vi "generate_avg.vi"(4 "Summed/Average":u16, 5 "C2 enabled":bool=TRUE caption="Enabled?", 6 "Trace numer":i32=1, 7 "C1 enabled":bool=TRUE caption="Enabled?", 11 "scope Q data":T1) -> ()   [LabVIEW 2023]
uses:
  <vilib>/Waveform/WDTOps.llb/WDT Align Waveform Timestamps DBL.vi
  <vilib>/Waveform/WDTFileIO.llb/Export Waveform To Spreadsheet File.vi
  <vilib>/regexp/Match Regular Expression.xnode
panel:
  out "Channel 2 summed":waveform(dbl)(graph)
  in  "waveforms out 2":waveform(dbl)[](array[waveform])
  out "Channel 2 RT avg":waveform(dbl)(graph)
  out "Channel 1 summed":waveform(dbl)(graph)
  out "Channel 1 RT avg":waveform(dbl)(graph)
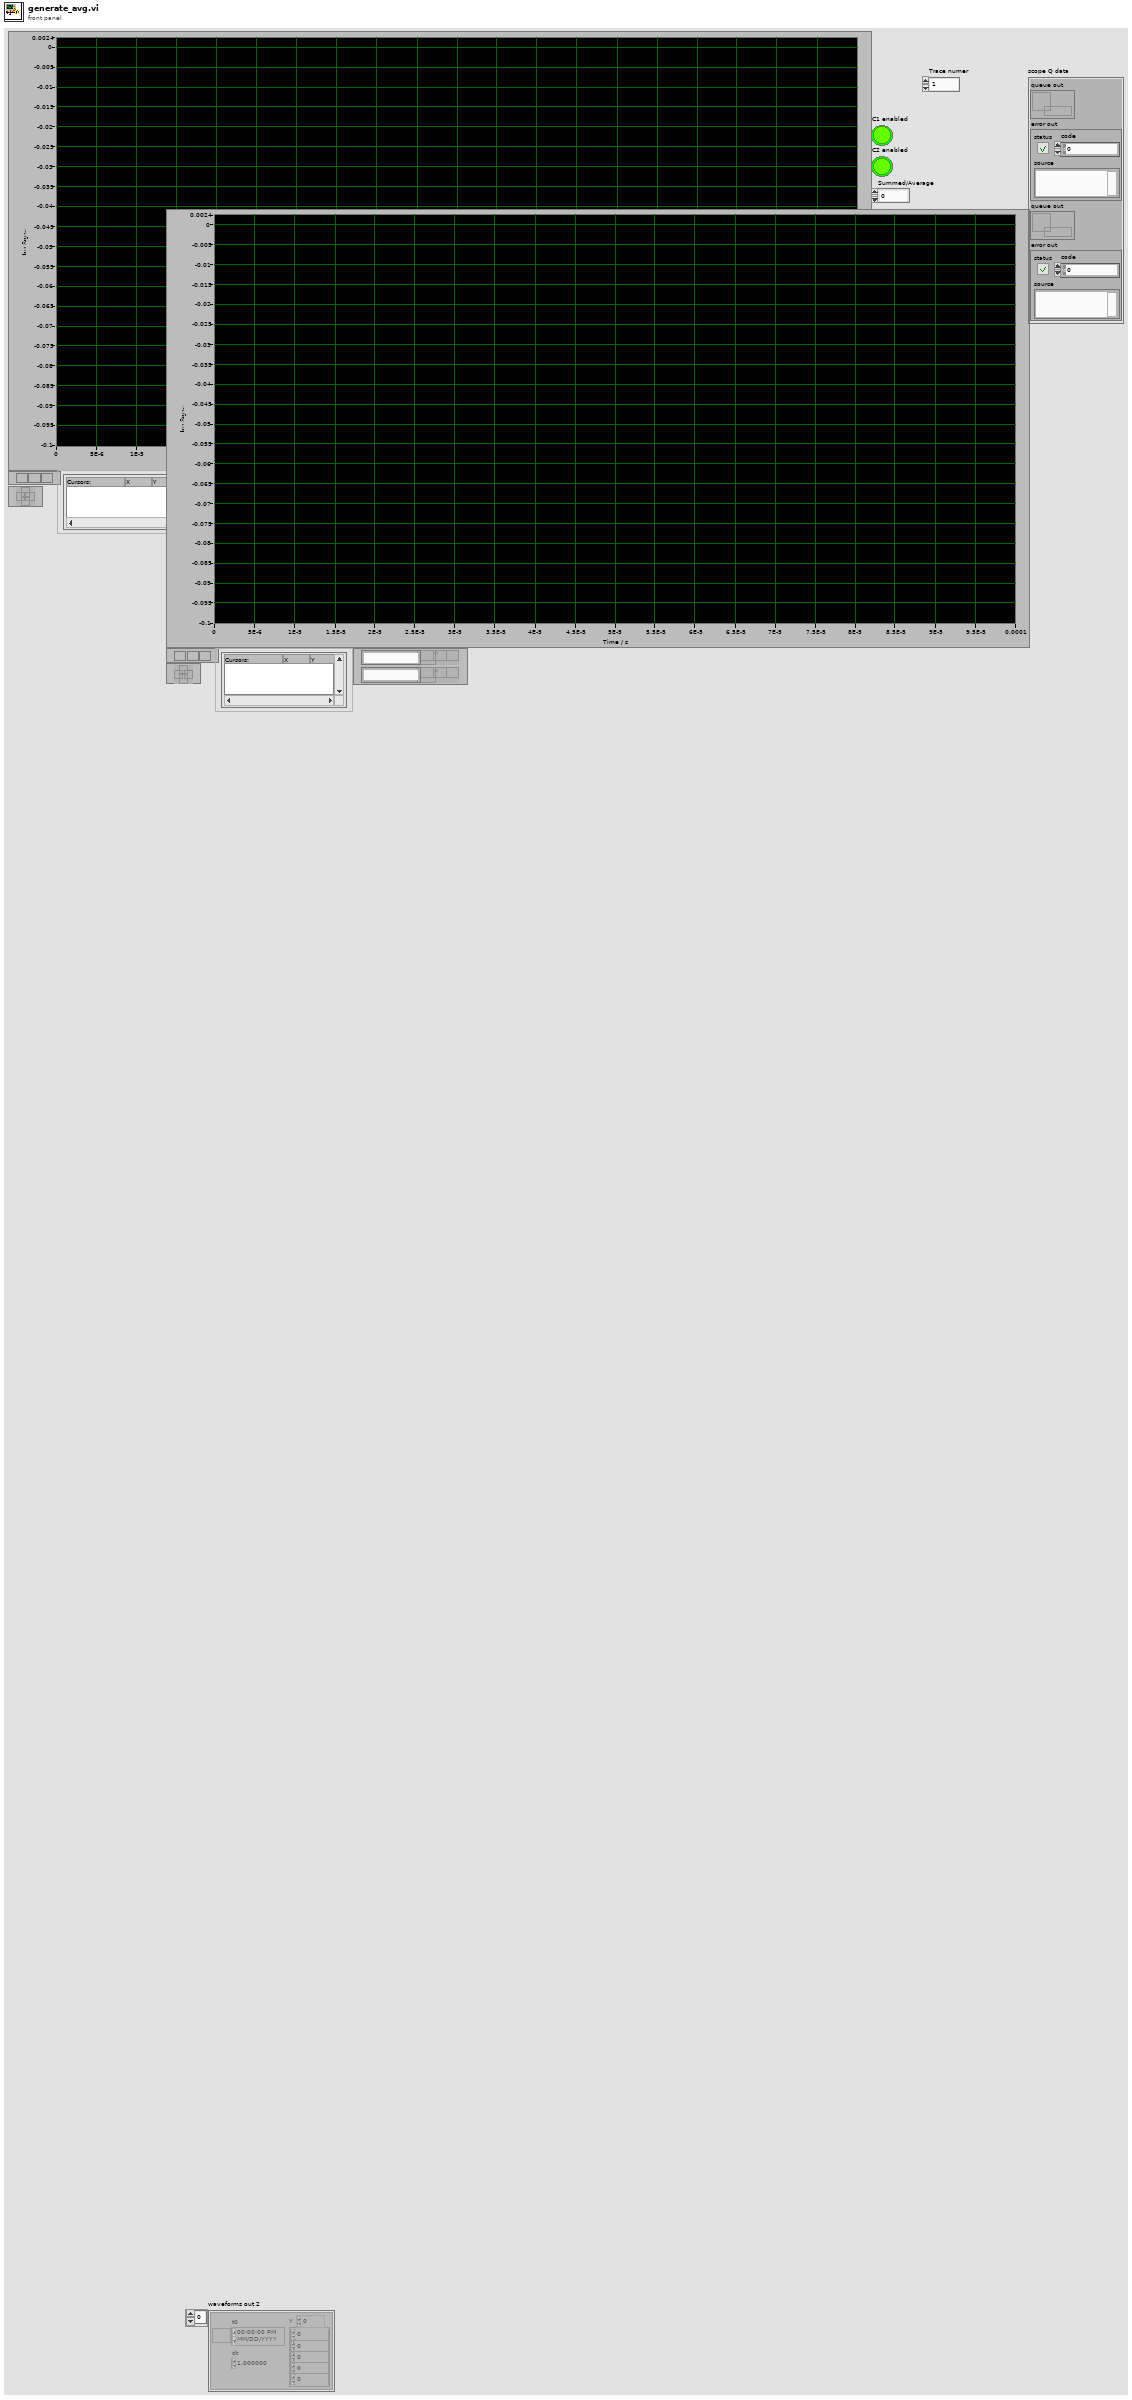
[diagram p1: front panel]
types:
  T1 = cluster{"queue out":refnum<queue>, "error out":errorcluster, "queue out":refnum<queue>, "error out":errorcluster}
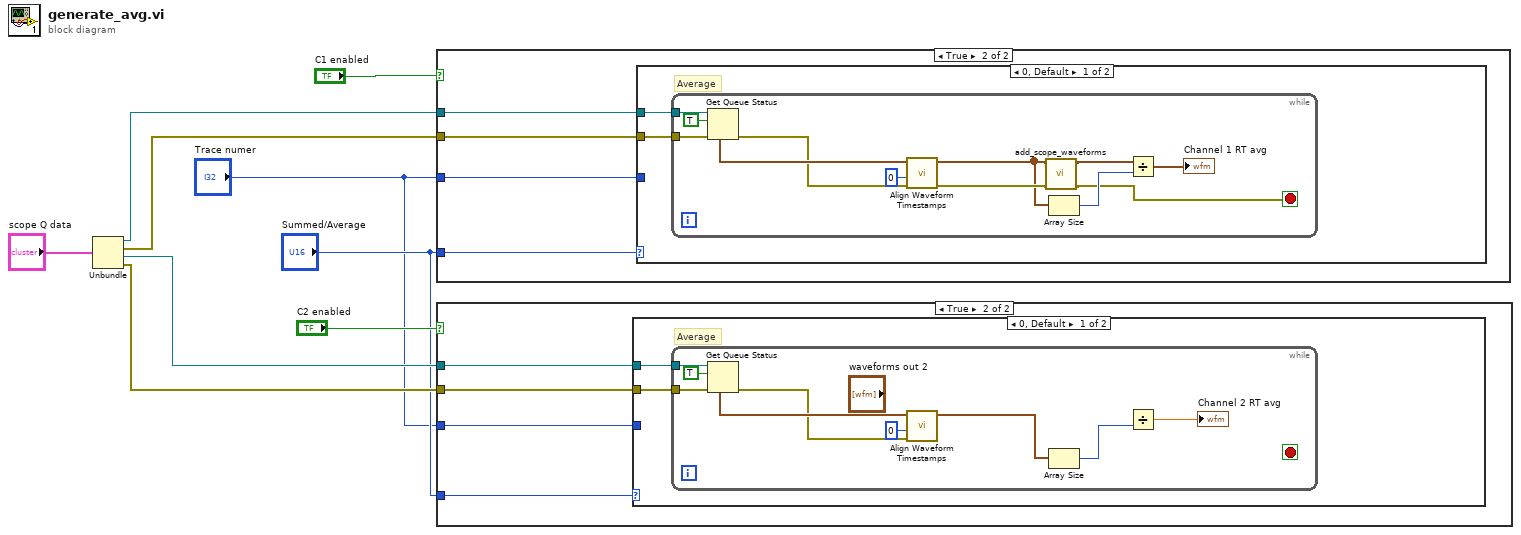
[diagram p0: block diagram]
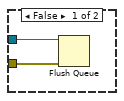
[diagram p2: hidden frame]
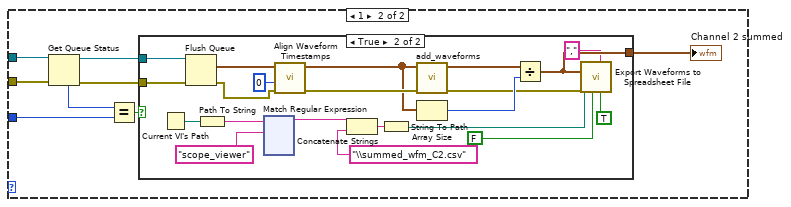
[diagram p3: hidden frame]
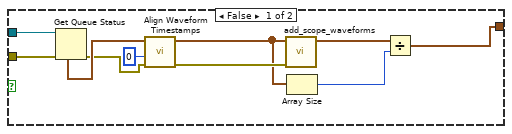
[diagram p4: hidden frame]
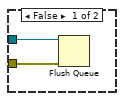
[diagram p5: hidden frame]
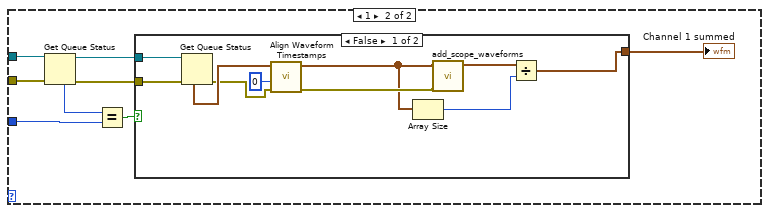
[diagram p6: hidden frame]
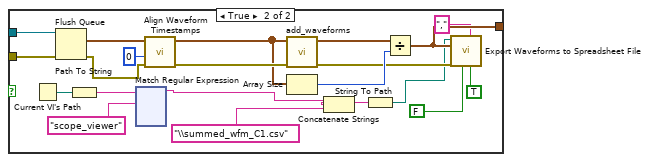
[diagram p7: hidden frame]
diagram:
  n1 = Unbundle("scope Q data") -> ("queue out"=w8:refnum<queue>, "error out"=w7:errorcluster, "queue out"=w6:refnum<queue>, "error out"=w5:errorcluster)
  n2 = case shown="True" "C1 enabled" {
    tunnel: w8 -> [w11 w14]
    tunnel: w7 -> [w10 w13]
    tunnel: "Summed/Average" -> [_ w15]
    tunnel: "Trace numer" -> [_ w12]
    frame False {
      n3 = Flush Queue(queue=w11, error in (no error)=w10) -> ()  [unwired: 3 out]
    }
    frame True {
      n4 = case shown="0, Default" w15 {
        tunnel: w14 -> [w17 w36]
        tunnel: w13 -> [w16 w37]
        tunnel: w12 -> [_ w30]
        frame 0, Default {
          # "Average"
          n5 = while {
            tunnel: w17 -> [w29]
            tunnel: w16 -> [w28]
            stop <- w20 stop-if-true
            n6 = Get Queue Status(queue=w29, return elements? (F)=TRUE, error in (no error)=w28) -> (error out=w26:errorcluster, elements=w27:waveform(dbl)[])  [unwired: 6 out]
            n7 = call-poly <vilib>:"Align Waveform Timestamps.vi"("error in (no error)"=w26, "index"=0, "waveforms in"=w27) -> ("error out"=w21:errorcluster, "waveforms out"=w18:waveform(dbl)[])  [unwired: 7 in]
            n8 = call "add_scope_waveforms.vi"("Error in (no error)"=w21, "Waveform array"=w18) -> ("Error out"=w20:errorcluster, "Summed waveform"=w19:waveform(dbl))  [unwired: 8 in]
            n9 = Array Size(array=w18) -> (size(s)=w24:i32)
            n10 = Divide(x=w19, y=w24) -> (x/y=→"Channel 1 RT avg":waveform(dbl))
          }
        }
        frame 1 {
          n11 = Get Queue Status(queue=w36, error in (no error)=w37) -> (queue out=w33:refnum<queue>, error out=w32:errorcluster, # elements in queue=w34:i32)  [unwired: 1 in, 5 out]
          n12 = Equal?(x=w34, y=w30) -> (x = y?=w35:bool)
          n13 = case shown="False" w35 {
            tunnel: w33 -> [w47 w68]
            tunnel: w32 -> [w46 w67]
            tunnel: [w41 w53] -> w31
            frame False {
              n14 = Get Queue Status(queue=w47, error in (no error)=w46) -> (error out=w42:errorcluster, elements=w43:waveform(dbl)[])  [unwired: 1 in, 6 out]
              n15 = call-poly <vilib>:"Align Waveform Timestamps.vi"("error in (no error)"=w42, "index"=0, "waveforms in"=w43) -> ("error out"=w40:errorcluster, "waveforms out"=w39:waveform(dbl)[])  [unwired: 7 in]
              n16 = Array Size(array=w39) -> (size(s)=w44:i32)
              n17 = call "add_scope_waveforms.vi"("Error in (no error)"=w40, "Waveform array"=w39) -> ("Summed waveform"=w38:waveform(dbl))  [unwired: 8 in, 1 out]
              n18 = Divide(x=w38, y=w44) -> (x/y=w41:waveform(dbl))
            }
            frame True {
              n19 = Current VI's Path() -> (path=w59:path)
              n20 = Flush Queue(queue=w68, error in (no error)=w67) -> (remaining elements=w63:waveform(dbl)[], error out=w60:errorcluster)  [unwired: 1 out]
              n21 = Path To String(path=w59) -> (string=w50:string)
              n22 = xnode "Match Regular Expression"("input string"=w50, "regular expression"="scope_viewer") -> ("before match"=w48:string)  [unwired: 4 in, 4 out]
              n23 = call-poly <vilib>:"Align Waveform Timestamps.vi"("error in (no error)"=w60, "index"=0, "waveforms in"=w63) -> ("error out"=w66:errorcluster, "waveforms out"=w65:waveform(dbl)[])  [unwired: 7 in]
              n24 = call "add_waveforms.vi"("Error in (no error)"=w66, "Waveform array"=w65) -> ("Error out"=w55:errorcluster, "Summed waveform"=w62:waveform(dbl))  [unwired: 8 in]
              n25 = Array Size(array=w65) -> (size(s)=w61:i32)
              n26 = Concatenate Strings(w48, "\\summed_wfm_C1.csv" ("string")) -> (w58:string)
              n27 = String To Path(string=w58) -> (path=w51:path)
              n28 = Divide(x=w62, y=w61) -> (x/y=w53:waveform(dbl))
              n29 = call-poly <vilib>:"Export Waveforms to Spreadsheet File.vi"("header? (write header:T)"=TRUE, "delimiter (Tab)"=",", "append to file? (new file:F)"=FALSE, "error in (no error)"=w55, "waveform"=w53, "file path (dialog if empty)"=w51) -> ()  [unwired: 4 in, 2 out]
            }
          }
          "Channel 1 summed" <- w31
        }
      }
    }
  }
  n30 = case shown="True" "C2 enabled" {
    tunnel: w6 -> [w187 w190]
    tunnel: w5 -> [w186 w189]
    tunnel: "Summed/Average" -> [_ w191]
    tunnel: "Trace numer" -> [_ w188]
    frame False {
      n31 = Flush Queue(queue=w187, error in (no error)=w186) -> ()  [unwired: 3 out]
    }
    frame True {
      n32 = case shown="0, Default" w191 {
        tunnel: w190 -> [w193 w212]
        tunnel: w189 -> [w192 w213]
        tunnel: w188 -> [_ w206]
        frame 0, Default {
          # "Average"
          n33 = while {
            tunnel: w193 -> [w205]
            tunnel: w192 -> [w204]
            stop <- w196 stop-if-true
            n34 = Get Queue Status(queue=w205, return elements? (F)=TRUE, error in (no error)=w204) -> (error out=w202:errorcluster, elements=w203:waveform(dbl)[])  [unwired: 6 out]
            n35 = call-poly <vilib>:"Align Waveform Timestamps.vi"("error in (no error)"=w202, "index"=0, "waveforms in"=w203) -> ("error out"=w201:errorcluster, "waveforms out"=w198:waveform(dbl)[])  [unwired: 7 in]
            n36 = Array Size(array=w198) -> (size(s)=w197:i32)
            n37 = Divide(y=w197) -> (x=w199:i32, x/y=→"Channel 2 RT avg":dbl)
          }
        }
        frame 1 {
          n38 = Get Queue Status(queue=w212, error in (no error)=w213) -> (queue out=w209:refnum<queue>, error out=w208:errorcluster, # elements in queue=w210:i32)  [unwired: 1 in, 5 out]
          n39 = Equal?(x=w210, y=w206) -> (x = y?=w211:bool)
          n40 = case shown="True" w211 {
            tunnel: w209 -> [w223 w244]
            tunnel: w208 -> [w222 w243]
            tunnel: [w217 w229] -> w207
            frame False {
              n41 = Get Queue Status(queue=w223, error in (no error)=w222) -> (error out=w218:errorcluster, elements=w219:waveform(dbl)[])  [unwired: 1 in, 6 out]
              n42 = call-poly <vilib>:"Align Waveform Timestamps.vi"("error in (no error)"=w218, "index"=0, "waveforms in"=w219) -> ("error out"=w216:errorcluster, "waveforms out"=w215:waveform(dbl)[])  [unwired: 7 in]
              n43 = call "add_scope_waveforms.vi"("Error in (no error)"=w216, "Waveform array"=w215) -> ("Summed waveform"=w214:waveform(dbl))  [unwired: 8 in, 1 out]
              n44 = Array Size(array=w215) -> (size(s)=w220:i32)
              n45 = Divide(x=w214, y=w220) -> (x/y=w217:waveform(dbl))
            }
            frame True {
              n46 = Current VI's Path() -> (path=w228:path)
              n47 = Flush Queue(queue=w244, error in (no error)=w243) -> (remaining elements=w239:waveform(dbl)[], error out=w236:errorcluster)  [unwired: 1 out]
              n48 = Path To String(path=w228) -> (string=w227:string)
              n49 = xnode "Match Regular Expression"("input string"=w227, "regular expression"="scope_viewer") -> ("before match"=w225:string)  [unwired: 4 in, 4 out]
              n50 = call-poly <vilib>:"Align Waveform Timestamps.vi"("error in (no error)"=w236, "index"=0, "waveforms in"=w239) -> ("error out"=w242:errorcluster, "waveforms out"=w241:waveform(dbl)[])  [unwired: 7 in]
              n51 = Concatenate Strings(w225, "\\summed_wfm_C2.csv" ("string")) -> (w235:string)
              n52 = String To Path(string=w235) -> (path=w233:path)
              n53 = call "add_waveforms.vi"("Error in (no error)"=w242, "Waveform array"=w241) -> ("Error out"=w231:errorcluster, "Summed waveform"=w238:waveform(dbl))  [unwired: 8 in]
              n54 = Array Size(array=w241) -> (size(s)=w237:i32)
              n55 = Divide(x=w238, y=w237) -> (x/y=w229:waveform(dbl))
              n56 = call-poly <vilib>:"Export Waveforms to Spreadsheet File.vi"("header? (write header:T)"=TRUE, "delimiter (Tab)"=",", "append to file? (new file:F)"=FALSE, "error in (no error)"=w231, "waveform"=w229, "file path (dialog if empty)"=w233) -> ()  [unwired: 4 in, 2 out]
            }
          }
          "Channel 2 summed" <- w207
        }
      }
    }
  }
